vi "exnSpectralBlock clear array phases.vi"(1 "phases in":cluster{"f0":dbl, "df":dbl, "phase":dbl[]}[](array[cluster]) {"phase" format="%.2p"; "f0" format="%.2p"; "df" format="%.2p"}) -> (0 "phases out":cluster{"f0":dbl, "df":dbl, "phase":dbl[]}[](array[cluster]) {"phase" format="%.2p"; "f0" format="%.2p"; "df" format="%.2p"})   [LabVIEW 2017]
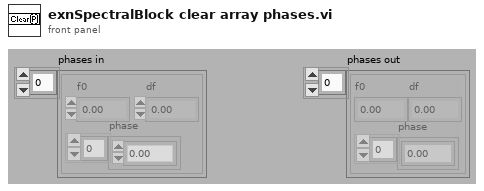
[diagram p1: front panel]
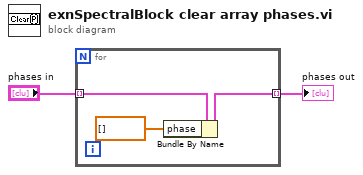
[diagram p0: block diagram]
diagram:
  n1 = for {
    tunnel: "phases in" -> [w4] mode=indexing
    tunnel: [w3] -> w1 mode=indexing
    n2 = Bundle By Name(cluster=w4, "phase"=dbl[] [] ("magnitude")) -> (w3:cluster{"f0":dbl, "df":dbl, "phase":dbl[]})
  }
  "phases out" <- w1
